vi "GetNI_BulkAcq.vi"(0 "Digitizer Settings":T8={"Digitizer delay (us) "=0.0, "rf points per line"=2048, "lines per plane"=128, "Samp Rate (Hz)"=100000000.0, "Additional dig delay (us)"=0.0, "Voltage Scale"=0.4, "Pre-Looks"=0, "Offset delay (us)"=0.0, "bits A/D"=8, "Avg Num"=1, "DigTimeOut"=5.0, "Rel Dig Delay"=0.0, "Dig Ch"=0, "LeCroyCluster"={"LeCroy Channels"=[TRUE, FALSE, FALSE, FALSE], "LC read pt offset"=0.0, "Sweep Avg"=FALSE}, "Main Digitizer"=enum."NI Digitizer", "Dig Config"=enum."Single channel", "Digitizer ID Cluster"={"Acqiris/Alazar/SP ID"=[], "NI Instr Handles"=[], "LeCroy VISA"="", "GaGe Handle"={"Handle"=0, "Sample size"=0, "Resolution"=0, "Offset"=0, "Channels"=0, "Boards"=0}, "ATS Ref"="ATS9350", "Acqiris Address"=["PCI::INSTR0"], "ADQRef"=refnum, "adq_cu_ptr"=refnum}, "Trigger Settings"={"Trig Source"=1, "Trig Coupling"=0, "Trig Slope"=0, "Level (mV)"=1500.0}, "Bulk Acq"=FALSE, "Bulk Start Indexes"=[], "Data Ref RF"=refnum, "NI ID/Channel"=[], "Total Dig CH"=1, "Xtra Ann Trig delay (us)"=10.0, "Fix Z Delay?"=FALSE, "One Way Transmission?"=FALSE, "Data Ref Log"=refnum} {"Trigger Settings"."Trig Slope" items=["Positive", "Negative"]; "Trigger Settings"."Level (mV)" format="%.2f"; "Trigger Settings"."Trig Coupling" items=["DC 1 MOhm", "AC 1 MOhm", "DC 50 Ohm", "AC 50 Ohm"]; "Trigger Settings"."Trig Source" items=["Chan 1", "External"]; "Rel Dig Delay" format="%.2f"; "DigTimeOut" format="%.2f"; "Avg Num" min=1; "Offset delay (us)" format="%.2f"; "Additional dig delay (us)" format="%.2f"; "Digitizer delay (us)" format="%.2f"}, 3 "NI Card":refnum<k15>, 4 "Ann Array Params":T1={"Synth Foc?"=FALSE, "Focal Zones"=41, "Switch T/R"=0, "Trans Geometry (mm)"={"Transducer"=0, "Geo Focus"=12.0, "a (radius)"=3.0, "# of rings"=5, "kerf space "=0.1, "Center Freq"=12.0}, "Sub Ap Excite?"=FALSE, "Full Array Scan?"=FALSE, "Xmt/Rcv"={"XMIT"=[TRUE, TRUE, TRUE, TRUE, TRUE], "RCV"=[TRUE, TRUE, TRUE, TRUE, TRUE]}, "PulseSpacing (us)"=0.0, "Xmit Ring"=0, "XMIT CHS"=0, "RCV CHS"=0, "GPU?"=FALSE, "Save TIFF?"=FALSE, "downfactor"=1, "RCV 1CH"=0} {"RCV 1CH" items=["All", "1", "2", "3", "4", "5"]; "Trans Geometry (mm)"."Transducer" items=["6D 12R 40 MHz"=0, "10D 31R 20 MHz"=1, "10D 23R 20 MHz"=2, "6D 23R 40 MHz"=3, "4.5D 10.7R 40 MHz"=4, "9D 23.5R 20 MHz"=5, "9D 25.8R 20MHz"=6, "Enter"=99]; "Switch T/R" min=1 max=5 step=1}, 6 "Motion Settings":T4={"No Motion?"=FALSE, "Motion System"=enum."NI 735x", "Motion Bd ID"=1, "Motion Profile"="SMAC1", "# Axis"=1, "Reverse Z axis?"=TRUE, "SMAC Axis"=0, "scan pair"=enum."y-(x) scan", "RT fps"=6.0, "Steps per mm"=[1000, 1000, 1000, 1000], "Motor Parameters"={"velocity ct/s"=[10000.0, 10000.0, 10000.0, 50000.0], "accel ct/s^2"=[50000.0, 50000.0, 50000.0, 200000.0]}, "One Way Scan"=FALSE, "Reverse One Way Scan"=FALSE, "Global Position (mm)"=[], "Plane"=0, "Distance between\nscan lines (um)"=0.0, "Distance between\nscan planes (um)"=0.0, "number of scan planes"=1, "Total steps in line"=0, "Xtra plane\ndistance  (um)"=100, "Xtra planes "=1, "Add Axis"=FALSE, "overshoot cts"=200, "BKPT Shift"=0, "Scan Start Time (ms)"=0, "ESP VISA"="GPIB::1::INSTR", "3rd Axis"=1, "GL Ref Out"=refnum, "Galil Address"=""} {"3rd Axis" items=["x", "y", "z", "w"]; "Xtra planes" min=1; "Xtra plane\ndistance  (um)" min=0; "Distance between\nscan planes (um)" format="%.2f"; "Distance between\nscan lines (um)" format="%.2f"; "SMAC Axis" items=["None"=0, "Axis 1"=1, "Axis 2"=2, "Axis 3"=3, "Axis 4"=4, "Axis 5"=5, "Axis 6"=6, "Axis 7"=7, "Axis 8"=8, "Vector Space 1"=17, "Vector Space 2"=18, "Vector Space 3"=19, "Vector Space 4"=20]; "Motion Bd ID" min=1 max=32 step=1}, 7 "errorin":errorcluster, 8 "File Array":string[](array[string]), 10 "lines per plane":i32, 15 "Reverse?":bool) -> (17 "Raw VGain (scale)":dbl, 18 "Gain Array":T12(array[cluster]), 21 "VGain (dB)":dbl, 27 "error out":errorcluster)   [LabVIEW 2022 SP3]
uses:
  -DigitizerRoutines/DigitizerSettings.ctl
  -DigitizerRoutines/Digitizer.ctl
  -DigitizerRoutines/DigConfig.ctl
  -DigitizerRoutines/DigitizerID.ctl
  C:/Windows/System32/ADQAPI_dotNet_helper.dll
  Motion Controllers/NI_controller/-NI_MotionRoutines/MotionParameters.ctl
  Motion Controllers/NI_controller/-NI_MotionRoutines/MotionSys.ctl
  Motion Controllers/-MotionRoutines/ScanAxis.ctl
  Motion Controllers/-MotionRoutines/3rdAxis.ctl
  Annular Array/-AnnularRoutines/AnnularArray.ctl
  Annular Array/-AnnularRoutines/TransGeometry.ctl
  Annular Array/-AnnularRoutines/ArrayGeometry.ctl
  <instrlib>/niScope/Acquire/Fetch/niScope Multi Fetch Binary 8.vi
  -ScanSystem/DataHandling/ReverseDataI8.vi
  Motion Controllers/-MotionRoutines/MotionGlobals.vi
panel:
  # "1-D and 2-D B scan settings"
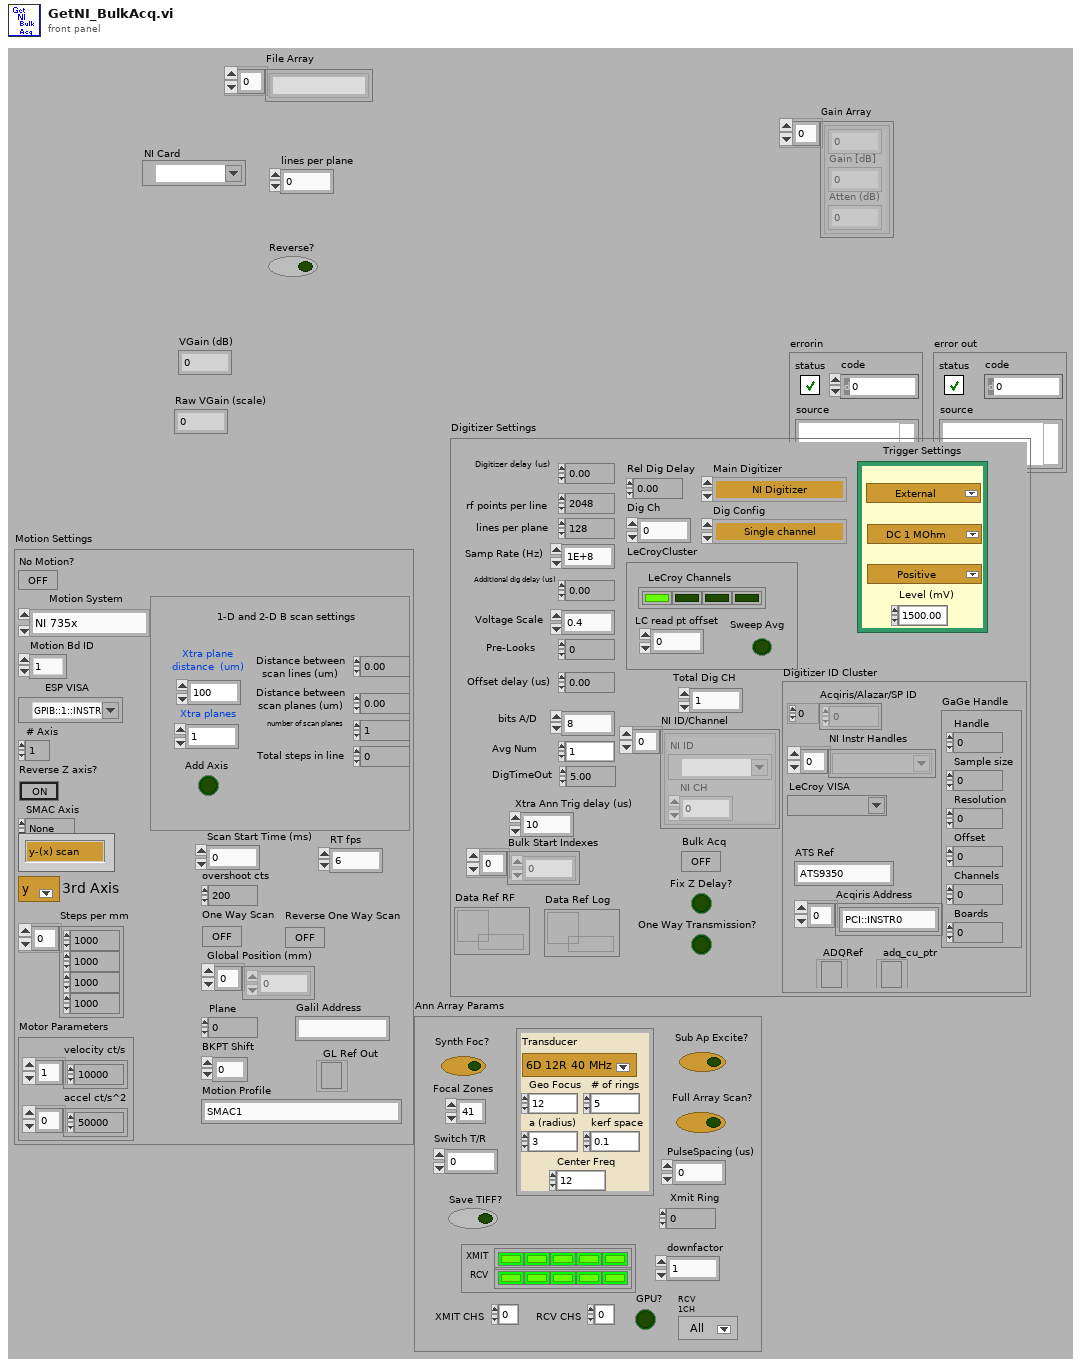
[diagram p1: front panel]
types:
  T1 = typedef "AnnularArray.ctl" = cluster{"Synth Foc?":bool, "Focal Zones":i16, "Switch T/R":i16, "Trans Geometry (mm)":T2, "Sub Ap Excite?":bool, "Full Array Scan?":bool, "Xmt/Rcv":cluster{"XMIT":bool[], "RCV":bool[]}, "PulseSpacing (us)":sgl, "Xmit Ring":i32, "XMIT CHS":u8, "RCV CHS":u8, "GPU?":bool, "Save TIFF?":bool, "downfactor":i32, "RCV 1CH":u16}
  T2 = typedef "TransGeometry.ctl" = cluster{"Transducer":T3, "Geo Focus":dbl, "a (radius)":dbl, "# of rings":i32, "kerf space ":dbl, "Center Freq":dbl}
  T3 = typedef "ArrayGeometry.ctl" = u16
  T4 = typedef "MotionParameters.ctl" = cluster{"No Motion?":bool, "Motion System":T5, "Motion Bd ID":u8, "Motion Profile":string, "# Axis":i8, "Reverse Z axis?":bool, "SMAC Axis":u16, "scan pair":T6, "RT fps":sgl, "Steps per mm":i32[], "Motor Parameters":cluster{"velocity ct/s":dbl[], "accel ct/s^2":dbl[]}, "One Way Scan":bool, "Reverse One Way Scan":bool, "Global Position (mm)":dbl[], "Plane":i32, "Distance between\nscan lines (um)":sgl, "Distance between\nscan planes (um)":sgl, "number of scan planes":i32, "Total steps in line":i32, "Xtra plane\ndistance  (um)":i32, "Xtra planes ":i32, "Add Axis":bool, "overshoot cts":i32, "BKPT Shift":i32, "Scan Start Time (ms)":u32, "ESP VISA":refnum<visa-resource-name>, "3rd Axis":T7, "GL Ref Out":refnum<k7>, "Galil Address":string}
  T5 = typedef "MotionSys.ctl" = enum16{"MM3000", "NI 735x", "Newport ESP", "No Motion Card", "Galil"}
  T6 = typedef "ScanAxis.ctl" = enum16{"y-(x) scan", "x-(y) scan", "z-(x) scan", "z-(y) scan", "y-(z) scan", "x-(z) scan", "w-(x) scan", "w-(y) scan", "w-(z) scan", "x-(w) scan", "y-(w) scan", "z-(w) scan"}
  T7 = typedef "3rdAxis.ctl" = u16
  T8 = typedef "DigitizerSettings.ctl" = cluster{"Digitizer delay (us) ":dbl, "rf points per line":i32, "lines per plane":i32, "Samp Rate (Hz)":dbl, "Additional dig delay (us)":dbl, "Voltage Scale":dbl, "Pre-Looks":i32, "Offset delay (us)":dbl, "bits A/D":i8, "Avg Num":i32, "DigTimeOut":sgl, "Rel Dig Delay":sgl, "Dig Ch":i32, "LeCroyCluster":cluster{"LeCroy Channels":bool[], "LC read pt offset":dbl, "Sweep Avg":bool}, "Main Digitizer":T9, "Dig Config":T10, "Digitizer ID Cluster":T11, "Trigger Settings":cluster{"Trig Source":u16, "Trig Coupling":u16, "Trig Slope":u16, "Level (mV)":dbl}, "Bulk Acq":bool, "Bulk Start Indexes":i32[], "Data Ref RF":refnum<data-value>, "NI ID/Channel":cluster{"NI ID":refnum<k15>, "NI CH":i32}[], "Total Dig CH":i32, "Xtra Ann Trig delay (us)":dbl, "Fix Z Delay?":bool, "One Way Transmission?":bool, "Data Ref Log":refnum<data-value>}
  T9 = typedef "Digitizer.ctl" = enum16{"Acqiris Digitizer", "NI Digitizer", "LeCroy", "GaGe", "AlazarTech", "No Digitizer", "Teledyne"}
  T10 = typedef "DigConfig.ctl" = enum16{"Single channel", "2 Chans w/ 2 Acqiris", "2 Chans w/ 1 Acqiris", "5-CH Pulser New", "5-CH pulser w/ ann array", "5-pass style ann array", "Empty"}
  T11 = typedef "DigitizerID.ctl" = cluster{"Acqiris/Alazar/SP ID":u32[], "NI Instr Handles":refnum<k15>[], "LeCroy VISA":refnum<visa-resource-name>, "GaGe Handle":cluster{"Handle":u32, "Sample size":u32, "Resolution":i32, "Offset":i32, "Channels":u32, "Boards":u32}, "ATS Ref":string, "Acqiris Address":string[], "ADQRef":refnum<k24>, "adq_cu_ptr":refnum<k24>}
  T12 = cluster{sgl, "Gain [dB]  ":sgl, "Atten (dB)":sgl}[]
  T13 = cluster{"actualSamples":i32, "absoluteInitialX":dbl, "relativeInitialX":dbl, "xIncrement":dbl, "offset":dbl, "gain":dbl, "reserved1":dbl, "reserved2":dbl}[]
  T14 = cluster{"actualSamples":i32, "absoluteInitialX":dbl, "relativeInitialX":dbl, "xIncrement":dbl, "offset":dbl, "gain":dbl, "reserved1":dbl, "reserved2":dbl}
  T15 = cluster{sgl, "Gain [dB]  ":sgl, "Atten (dB)":sgl}
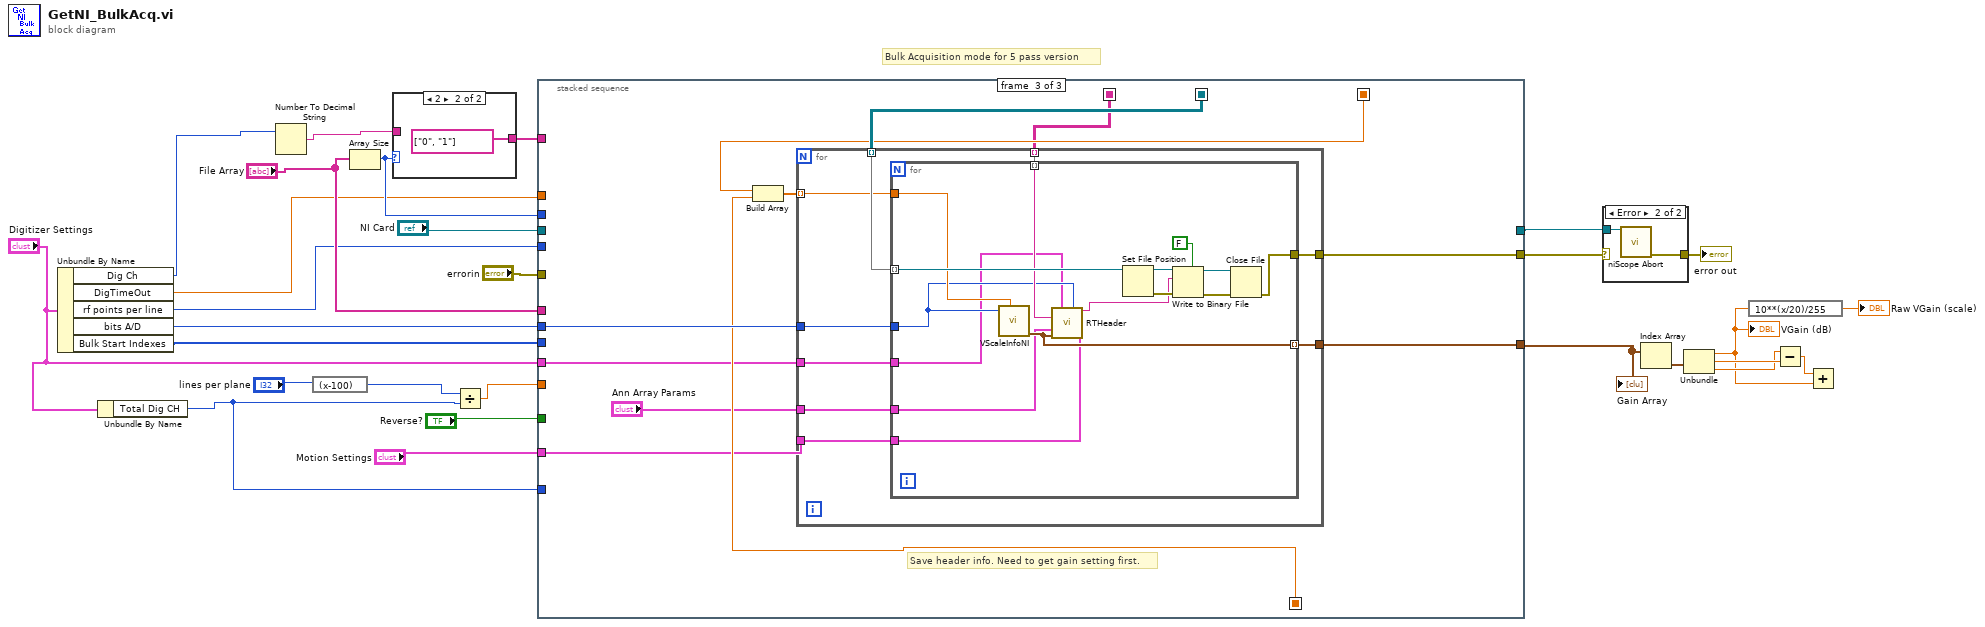
[diagram p0: block diagram]
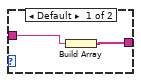
[diagram p2: hidden frame]
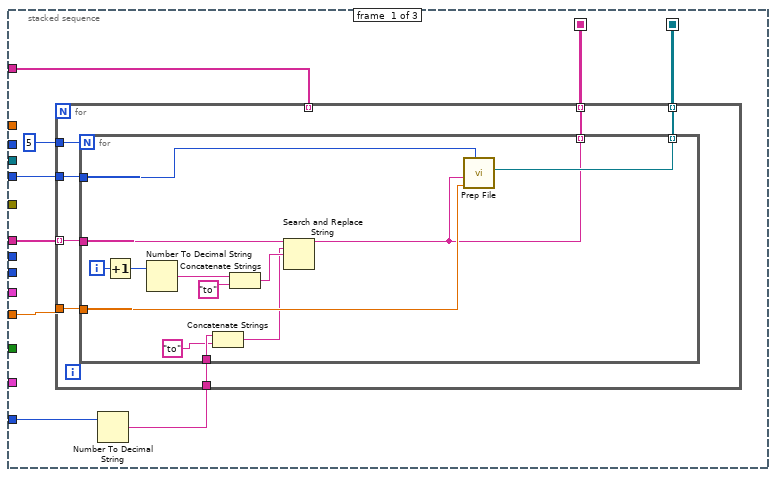
[diagram p3: hidden frame]
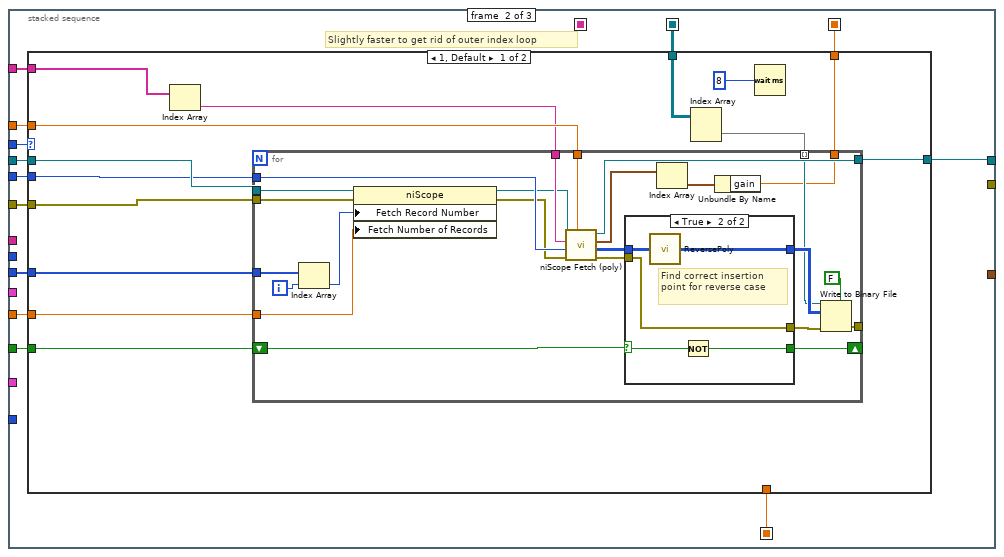
[diagram p4: hidden frame]
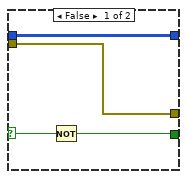
[diagram p5: hidden frame]
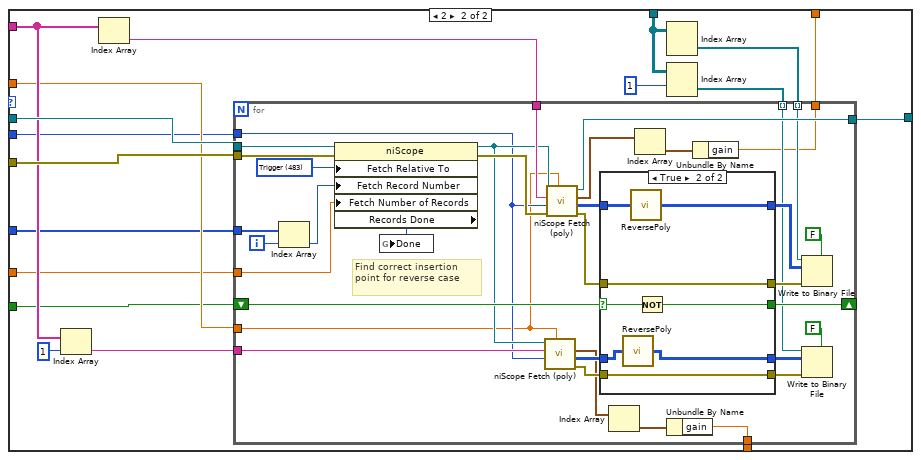
[diagram p6: hidden frame]
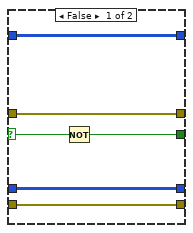
[diagram p7: hidden frame]
diagram:
  # "Bulk Acquisition mode for 5 pass version"
  n1 = Unbundle By Name("Digitizer Settings") -> ("Dig Ch"=w7:i32, "DigTimeOut"=w8:sgl, "rf points per line"=w9:i32, "bits A/D"=w10:i8, "Bulk Start Indexes"=w5:i32[])
  n2 = Unbundle By Name("Digitizer Settings") -> ("Total Dig CH"=w1:i32)
  n3 = Number To Decimal String(number=w7) -> (decimal integer string=w19:string)  [unwired: 1 out]
  n4 = expression code="(x-100)"("lines per plane") -> (w4:i32)
  n5 = Array Size(array="File Array") -> (size(s)=w20:i32)
  n6 = case shown="2" w20 {
    tunnel: [w30 string[] ["0", "1"] ("File Array")] -> w21
    tunnel: w19 -> [w29 _]
    frame Default {
      n7 = Build Array(w29) -> (w30:string[])
    }
    frame 2 {
    }
  }
  n8 = Divide(x=w4, y=w1) -> (x/y=w3:dbl)
  n9 = stacked-sequence {
    seq-local: [w39 _ _] -> [_ w69 w198]
    seq-local: [_ w63 _] -> [_ _ w196]
    seq-local: [_ w62 _] -> [_ _ w191]
    seq-local: [w34 _ _] -> [_ _ w193]
    tunnel: [_ w61 _] -> w12
    tunnel: [_ _ w194] -> w13
    tunnel: "NI Card" -> [_ w73 _]
    tunnel: w8 -> [_ w72 _]
    tunnel: w3 -> [w36 w67 _]
    tunnel: w21 -> [w40 w71 _]
    tunnel: w9 -> [w37 w70 _]
    tunnel: "File Array" -> [w38 _ _]
    tunnel: "errorin" -> [_ w68 _]
    tunnel: w20 -> [_ w66 _]
    tunnel: w5 -> [_ w65 _]
    tunnel: "Reverse?" -> [_ w64 _]
    tunnel: [_ _ w197] -> w14
    tunnel: w10 -> [_ _ w192]
    tunnel: "Digitizer Settings" -> [_ _ w190]
    tunnel: "Motion Settings" -> [_ _ w189]
    tunnel: w1 -> [w33 _ _]
    frame #0 {
      n10 = Number To Decimal String(number=w33) -> (decimal integer string=w32:string)  [unwired: 1 out]
      n11 = for {
        tunnel: w40 -> [_] mode=indexing
        tunnel: [w47] -> w39 mode=indexing
        tunnel: w38 -> [w46] mode=indexing
        tunnel: w37 -> [w45]
        tunnel: w36 -> [w44]
        tunnel: 5 -> [w43]
        tunnel: [w42] -> w34 mode=indexing
        tunnel: w32 -> [w41]
        n12 = for {
          N: w43 -> [_]
          tunnel: [w54] -> w47 mode=indexing
          tunnel: w46 -> [w56]
          tunnel: w45 -> [w53]
          tunnel: w44 -> [w52]
          tunnel: [w51] -> w42 mode=indexing
          tunnel: w41 -> [w50]
          i -> [w55]
          n13 = Increment(x=w55) -> (x+1=w57:i32)
          n14 = Number To Decimal String(number=w57) -> (decimal integer string=w58:string)  [unwired: 1 out]
          n15 = Concatenate Strings(w50, "to") -> (w48:string)
          n16 = Concatenate Strings(w58, "to") -> (w60:string)
          n17 = Search and Replace String(input string=w56, search string=w48, replace string=w60) -> (result string=w51:string)  [unwired: 2 in, 6 out]
          n18 = call "Prep File.vi"("Num Samps"=w53, "Num Segs"=w52, "File Name"=w51) -> ("refnum out"=w54:refnum<file>)  [unwired: 4 in, 1 out]
        }
      }
    }
    frame #1 {
      # "Slightly faster to get rid of outer index loop"
      n19 = case shown="1, Default" w66 {
        tunnel: [w79 w126] -> w61
        tunnel: w73 -> [w87 w136]
        tunnel: w72 -> [w86 w133]
        tunnel: w71 -> [w82 w135]
        tunnel: w70 -> [w85 w132]
        tunnel: w69 -> [w80 w130]
        tunnel: w68 -> [w84 w137]
        tunnel: w67 -> [w78 w128]
        tunnel: w65 -> [w77 w127]
        tunnel: w64 -> [w76 w125]
        tunnel: [w74 w122] -> w63
        tunnel: [_ w121] -> w62
        frame 1, Default {
          n20 = Index Array(array=w82) -> (element=w81:string)  [unwired: 1 in]
          n21 = Index Array(array=w80) -> (element=w75:refnum<file>[])  [unwired: 2 in]
          n22 = for {
            tunnel: [w111] -> w79
            tunnel: w81 -> [w110]
            tunnel: w86 -> [w109]
            tunnel: w84 -> [w101]
            tunnel: w85 -> [w105]
            tunnel: [w106] -> _
            tunnel: w87 -> [w103]
            tunnel: w78 -> [w100]
            shift-right: [w93] -> _
            shift-left: w76 -> [w97]
            tunnel: w77 -> [w96]
            tunnel: w75 -> [w92] mode=indexing
            tunnel: [w88] -> w74
            i -> [w95]
            n23 = Index Array(array=w96, index=w95) -> (element=w94:i32)
            n24 = property class="niScope"(reference=w103, error in=w101, "Fetch Record Number"=w94, "Fetch Number of Records"=w100) -> (reference out=w104:refnum<k15>, error out=w102:errorcluster)
            n25 = call-poly <instrlib>:"niScope Fetch (poly).vi"("timeout"=w109, "error in"=w102, "numSamples"=w105, "channels"=w110, "instrument handle"=w104) -> ("error out"=w98:errorcluster, "wfm"=w91:i8[][], "wfm info"=w90:T13, "instrument handle out"=w111:refnum<k15>)  [unwired: 3 out]
            n26 = case shown="True" w97 {
              selector: w97 -> [w113 w117]
              tunnel: [w115 w120] -> w108
              tunnel: w91 -> [w115 w119]
              tunnel: [w114 w118] -> w99
              tunnel: w98 -> [w114 w118]
              tunnel: [w112 w116] -> w93
              frame False {
                n27 = Not(x=w113) -> (.not. x?=w112:bool)
              }
              frame True {
                # "Find correct insertion point for reverse case"
                n28 = call-poly "ReversePoly.vi"("Array in"=w119) -> ("Array out"=w120:i8[][])
                n29 = Not(x=w117) -> (.not. x?=w116:bool)
              }
            }
            n30 = Index Array(array=w90) -> (element=w89:T14)  [unwired: 1 in]
            n31 = Unbundle By Name(w89) -> ("gain"=w88:dbl)
            n32 = Write to Binary File(file (use dialog)=w92, data=w108, error in=w99, 5:FALSE ("prepend array or string size? (T)")) -> (error out=w106:errorcluster)  [unwired: 1 in, 3 out]
          }
          n33 = Wait (ms)(milliseconds to wait=8) -> ()  [unwired: 1 out]
        }
        frame 2 {
          n34 = Index Array(array=w135, index=1) -> (element=w124:string)
          n35 = Index Array(array=w135) -> (element=w138:string)  [unwired: 1 in]
          n36 = Index Array(array=w130) -> (element=w131:refnum<file>[])  [unwired: 2 in]
          n37 = Index Array(array=w130, index (row)=1) -> (element=w123:refnum<file>[])  [unwired: 1 in]
          n38 = for {
            tunnel: [w173] -> w126
            tunnel: w138 -> [w172]
            tunnel: w133 -> [w152]
            tunnel: w137 -> [w165]
            tunnel: w132 -> [w153]
            tunnel: w131 -> [w145] mode=indexing
            tunnel: w136 -> [w167]
            tunnel: w128 -> [w164]
            shift-right: [w156] -> _
            shift-left: w125 -> [w161]
            tunnel: w127 -> [w159]
            tunnel: w124 -> [w155]
            tunnel: w123 -> [w146] mode=indexing
            tunnel: [w142] -> w122
            tunnel: [w139] -> w121
            i -> [w157]
            w168 = 483 items=["Start"=482, "Trigger"=483, "Pretrigger"=477, "Now"=481, "Read Pointer"=388] ("Fetch:Fetch Relative To")
            # "Find correct insertion point for reverse case"
            n39 = Index Array(array=w159, index=w157) -> (element=w158:i32)
            n40 = property class="niScope"(reference=w167, error in=w165, "Fetch Relative To"=w168, "Fetch Record Number"=w158, "Fetch Number of Records"=w164) -> (reference out=w154:refnum<k15>, error out=w166:errorcluster, "Records Done"=w160:i32)
            n41 = global write "MotionGlobals.vi" "Done"(w160) -> ()
            n42 = call-poly <instrlib>:"niScope Fetch (poly).vi"("timeout"=w152, "numSamples"=w153, "channels"=w155, "instrument handle"=w154) -> ("error out"=w147:errorcluster, "wfm"=w150:i8[][], "wfm info"=w140:T13)  [unwired: 1 in, 4 out]
            n43 = call-poly <instrlib>:"niScope Fetch (poly).vi"("timeout"=w152, "error in"=w166, "numSamples"=w153, "channels"=w172, "instrument handle"=w154) -> ("error out"=w162:errorcluster, "wfm"=w170:i8[][], "wfm info"=w143:T13, "instrument handle out"=w173:refnum<k15>)  [unwired: 3 out]
            n44 = case shown="True" w161 {
              selector: w161 -> [w177 w184]
              tunnel: [w179 w187] -> w171
              tunnel: w170 -> [w179 w186]
              tunnel: [w178 w185] -> w163
              tunnel: w162 -> [w178 w185]
              tunnel: [w176 w183] -> w156
              tunnel: [w175 w180] -> w149
              tunnel: w150 -> [w175 w181]
              tunnel: [w174 w182] -> w148
              tunnel: w147 -> [w174 w182]
              frame False {
                n45 = Not(x=w177) -> (.not. x?=w176:bool)
              }
              frame True {
                n46 = call-poly "ReversePoly.vi"("Array in"=w181) -> ("Array out"=w180:i8[][])
                n47 = call-poly "ReversePoly.vi"("Array in"=w186) -> ("Array out"=w187:i8[][])
                n48 = Not(x=w184) -> (.not. x?=w183:bool)
              }
            }
            n49 = Index Array(array=w140) -> (element=w141:T14)  [unwired: 1 in]
            n50 = Index Array(array=w143) -> (element=w144:T14)  [unwired: 1 in]
            n51 = Unbundle By Name(w141) -> ("gain"=w139:dbl)
            n52 = Unbundle By Name(w144) -> ("gain"=w142:dbl)
            n53 = Write to Binary File(file (use dialog)=w145, data=w171, error in=w163, 5:FALSE ("prepend array or string size? (T)")) -> ()  [unwired: 1 in, 4 out]
            n54 = Write to Binary File(file (use dialog)=w146, data=w149, error in=w148, 5:FALSE ("prepend array or string size? (T)")) -> ()  [unwired: 1 in, 4 out]
          }
        }
      }
    }
    frame #2 {
      # "Save header info. Need to get gain setting first."
      n55 = Build Array(w196, w191) -> (w195:dbl[])
      n56 = for {
        tunnel: w198 -> [w207] mode=indexing
        tunnel: [w206] -> w197
        tunnel: w195 -> [w205] mode=indexing
        tunnel: [w204] -> w194
        tunnel: w193 -> [w203] mode=indexing
        tunnel: w192 -> [w202]
        tunnel: w190 -> [w201]
        tunnel: w189 -> [w200]
        tunnel: "Ann Array Params" -> [w199]
        n57 = for {
          tunnel: w207 -> [w219] mode=indexing
          tunnel: [w217] -> w206 mode=indexing
          tunnel: w205 -> [w216]
          tunnel: [w213] -> w204
          tunnel: w203 -> [w212] mode=indexing
          tunnel: w202 -> [w211]
          tunnel: w201 -> [w210]
          tunnel: w200 -> [w209]
          tunnel: w199 -> [w208]
          n58 = call "VScaleInfoNI.vi"("A/D bits"=w211, "gain"=w216) -> ("Voltage Scale"=w217:T15)  [unwired: 5 in, 3 out]
          n59 = call "RTHeader.vi"("Digitizer Settings"=w210, "Dig Word Size"=w211, "File Name In"=w212, "Ann Array Params"=w208, "Votage scaling"=w217, "Motion Settings"=w209) -> ("Header String Out"=w221:string)  [unwired: 8 in, 1 out]
          n60 = Set File Position(refnum=w219) -> (refnum out=w220:refnum<file>, error out=w222:errorcluster)  [unwired: 3 in]
          n61 = Write to Binary File(file (use dialog)=w220, data=w221, error in=w222, 5:FALSE ("prepend array or string size? (T)")) -> (refnum out=w218:refnum<file>, error out=w214:errorcluster)  [unwired: 2 in, 1 out]
          n62 = Close File(refnum=w218, error in=w214) -> (error out=w213:errorcluster)  [unwired: 1 out]
        }
      }
    }
  }
  "Gain Array" <- w14
  n63 = case shown="Error" w13 {
    selector: w13 -> [w223 _]
    tunnel: w12 -> [_ w225]
    tunnel: [w223 w224] -> w22
    frame No Error {
    }
    frame Error {
      n64 = call <instrlib>:"niScope Abort.vi"("instrument handle"=w225) -> ("error out"=w224:errorcluster)  [unwired: 1 in, 13 out]
    }
  }
  "error out" <- w22
  n65 = Index Array(array=w14) -> (element=w23:T15)  [unwired: 1 in]
  n66 = Unbundle(w23) -> (w24:sgl, "Gain [dB]"=w26:sgl, "Atten (dB)"=w25:sgl)
  "VGain (dB)" <- w24
  n67 = expression code="10**(x/20)/255"(w24) -> (→"Raw VGain (scale)":sgl)
  n68 = Subtract(x=w25, y=w26) -> (x-y=w27:sgl)
  n69 = Add(x=w27, y=w24) -> ()  [unwired: 1 out]
